vi "PPMSDR - Continuous IV.vi"() -> ()   [LabVIEW 2013]
panel:
  in  "stop":bool
  in  "Experiment folder name":string="02-IV test"
  in  "Notes":string="Seems lead 1 has the large barrier, while lead 28 is about the same (slightly better) than 27.\nVbg=-0.66V\n\nI1=Rightwire 2/27  5mVac, 0.2, sawtooth wave\nV1: 4-terminal left wire 3/5\nV2:  cross wire 4/28\n"
  in  "Target B field":dbl
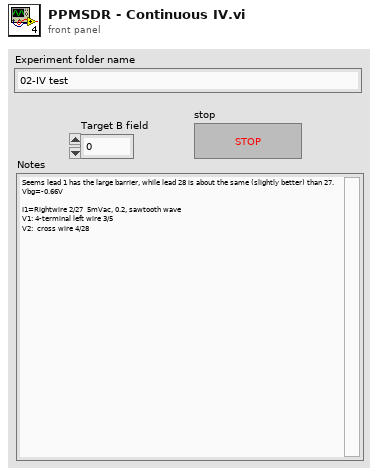
[diagram p1: front panel]
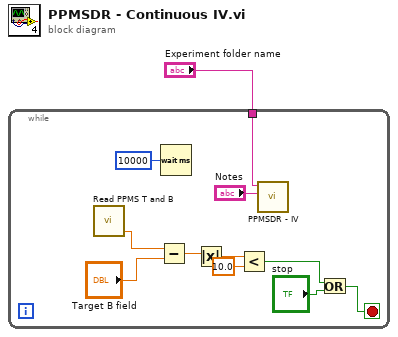
[diagram p0: block diagram]
diagram:
  n1 = while {
    tunnel: "Experiment folder name" -> [w5]
    stop <- w2 stop-if-true
    n2 = call <userlib>:"Read PPMS T and B.vi"() -> ("Field"=w11:dbl)  [unwired: 3 in, 2 out]
    n3 = Subtract(x=w11, y="Target B field") -> (x-y=w9:dbl)
    n4 = Wait (ms)(milliseconds to wait=u32 10000) -> ()  [unwired: 1 out]
    n5 = Absolute Value(x=w9) -> (abs(x)=w8:dbl)
    n6 = Less?(x=w8, y=10.0) -> (x < y?=w4:bool)
    n7 = call "PPMSDR - IV.vi"("Notes"="Notes", "Experiment folder name"=w5) -> ()  [unwired: 10 in]
    n8 = Or(x=w4, y="stop") -> (x .or. y?=w2:bool)
  }
